vi "Initialize.vi"(8 "error in":errorcluster, 11 "Client in":refnum<class "Client.lvclass">) -> (0 "error out":errorcluster, 3 "Client out":refnum<class "Client.lvclass">)   [LabVIEW 2014, in "Client.lvclass"]
uses:
  Client.lvclass
  Topic_class/Topic.lvclass
  Client.lvclass/Client.ctl
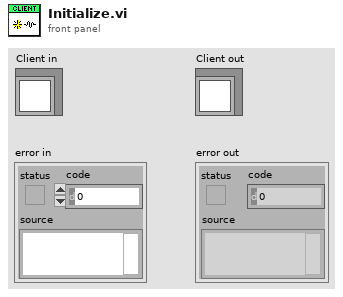
[diagram p1: front panel]
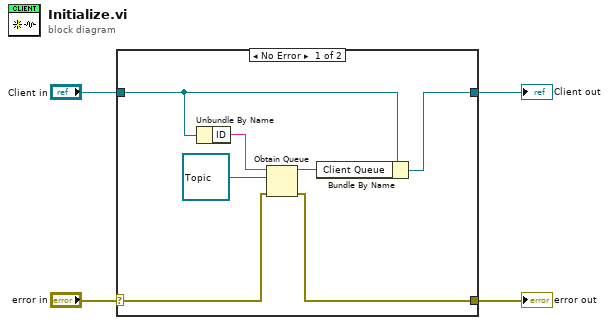
[diagram p0: block diagram]
diagram:
  n1 = case shown="No Error" "error in" {
    selector: "error in" -> [w8 w13]
    tunnel: [w7 w13] -> w3
    tunnel: [w5 w12] -> w1
    tunnel: "Client in" -> [w6 w12]
    frame No Error {
      n2 = Unbundle By Name(w6) -> ("ID"=w11:string)
      n3 = Obtain Queue(name (unnamed)=w11, element data type=refnum<class "Topic.lvclass"> refnum ("Topic.lvclass"), error in (no error)=w8) -> (queue out=w9:refnum<queue>, error out=w7:errorcluster)  [unwired: 2 in, 1 out]
      n4 = Bundle By Name(cluster=w6, "Client Queue"=w9) -> (w5:refnum<class "Client.lvclass">)
    }
    frame Error {
    }
  }
  "error out" <- w3
  "Client out" <- w1
